vi "Lift Manager.vi"(1 "Setpoint":dbl) -> (0 "Current Height":dbl)   [LabVIEW 2014]
uses:
  <vilib>/Rock Robotics/Network Tables/SD Read Numeric Array.vi
  <vilib>/Rock Robotics/Network Tables/SD Write Boolean.vi
  <vilib>/addons/control/pid/pid.llb/PID (DBL).vi
  <vilib>/addons/control/pid/NI_PID_pid.lvlib
  <vilib>/ptbypt/NI_PtbyPt.lvlib
panel:
  out "Encoder Value":dbl
  in  "Zero Encoder":bool
  in  "Disabled?":bool=TRUE
  out "Motor":dbl
  out "Waveform Chart":cluster{"Distance":dbl, "output":dbl}(graph)
  in  "PID gains Down":T1={"proportional gain (Kc)"=2.0, "integral time (Ti, min)"=0.0, "derivative time (Td, min)"=0.0}
  in  "PID gains UP":T1={"proportional gain (Kc)"=2.0, "integral time (Ti, min)"=0.0, "derivative time (Td, min)"=0.0}
  # "Max: 24"
  # "Min: 8"
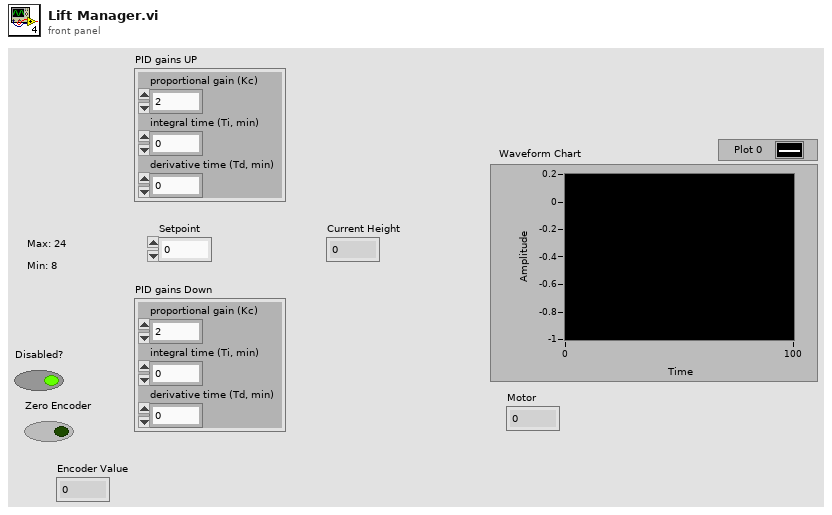
[diagram p1: front panel]
types:
  T1 = cluster{"proportional gain (Kc)":dbl, "integral time (Ti, min)":dbl, "derivative time (Td, min)":dbl}
  T2 = typedef "WPI_DigitalInputDevRef.ctl" = cluster{"DevStatus":errorcluster, "DIO Channel":T3, "Controller":T4}
  T3 = typedef "FPGA_DIOChannel.ctl" = enum8{"DIO 0", "DIO 1", "DIO 2", "DIO 3", "DIO 4", "DIO 5", "DIO 6", "DIO 7", "DIO 8", "DIO 9", "DIO MXP 0", "DIO MXP 1", "DIO MXP 2", "DIO MXP 3", "DIO MXP 4", "DIO MXP 5", "DIO MXP 6", "DIO MXP 7", "DIO MXP 8", "DIO MXP 9", "DIO MXP 10", "DIO MXP 11", "DIO MXP 12", "DIO MXP 13", "DIO MXP 14", "DIO MXP 15", "Invalid"}
  T4 = typedef "FPGA_TypedefDigitalModule.ctl" = enum16{"Controller 1"}
  T5 = typedef "WPI_EncoderDevRef.ctl" = cluster{"DevStatus":errorcluster, "EncoderIndex":T6, "CounterIndex":T7, "DistancePerCount":dbl, "Decoding Type":T8}
  T6 = typedef "FPGA_EncoderIdx.ctl" = enum8{"Enc 0", "Enc 1", "Enc 2", "Enc 3", "Enc 4", "Enc 5", "Enc 6", "Enc 7", "Invalid"}
  T7 = typedef "FPGA_CounterCtrSystemIndex.ctl" = enum8{"Ctr 0", "Ctr 1", "Ctr 2", "Ctr 3", "Ctr 4", "Ctr 5", "Ctr 6", "Ctr 7", "Invalid"}
  T8 = typedef "WPI_EncoderType.ctl" = enum16{"1x", "2x", "4x"}
  T9 = typedef "WPI_MotorControlDeviceRef.ctl" = cluster{"DeviceStatus":errorcluster, "Type":T10, "PWM":cluster{"Controller":T4, "PWM Channel":T11, "DeadBand":T12}, "CAN":cluster{"Device Number":u8, "Control Mode":T13, "Semaphore":T14, "Max Vout":dbl, "TalonSRX Control Mode":T15}, "Invert":bool, "TransformRef":T16, "InvTransformRef":T16}
  T10 = typedef "WPI_MotorControlType.ctl" = enum16{"PWM", "CAN", "CANTalonSRX"}
  T11 = typedef "FPGA_DIOPWMChannel.ctl" = enum8{"PWM 0", "PWM 1", "PWM 2", "PWM 3", "PWM 4", "PWM 5", "PWM 6", "PWM 7", "PWM 8", "PWM 9", "PWM MXP 0", "PWM MXP 1", "PWM MXP 2", "PWM MXP 3", "PWM MXP 4", "PWM MXP 5", "PWM MXP 6", "PWM MXP 7", "PWM MXP 8", "PWM MXP 9", "Invalid"}
  T12 = typedef "WPI_PWMDeadband.ctl" = cluster{"Name":string, "maxPositivePwm":i32, "minPositivePwm":i32, "centerPwm":i32, "maxNegativePwm":i32, "minNegativePwm":i32, "angularRange":u16}
  T13 = typedef "WPI_CANJaguar_ControlMode.ctl" = enum8{"Percent VBus", "Current", "Speed", "Position", "Voltage"}
  T14 = typedef "Semaphore RefNum" = refnum<k1>
  T15 = typedef "WPI_CANTalonSRX_APIControlMode.ctl" = enum8{"Percent VBus", "Speed", "Position", "Slave", "Unchanged / Invalid"}
  T16 = typedef "WPI_PWMTransform_ConPane.ctl" = refnum<vi>
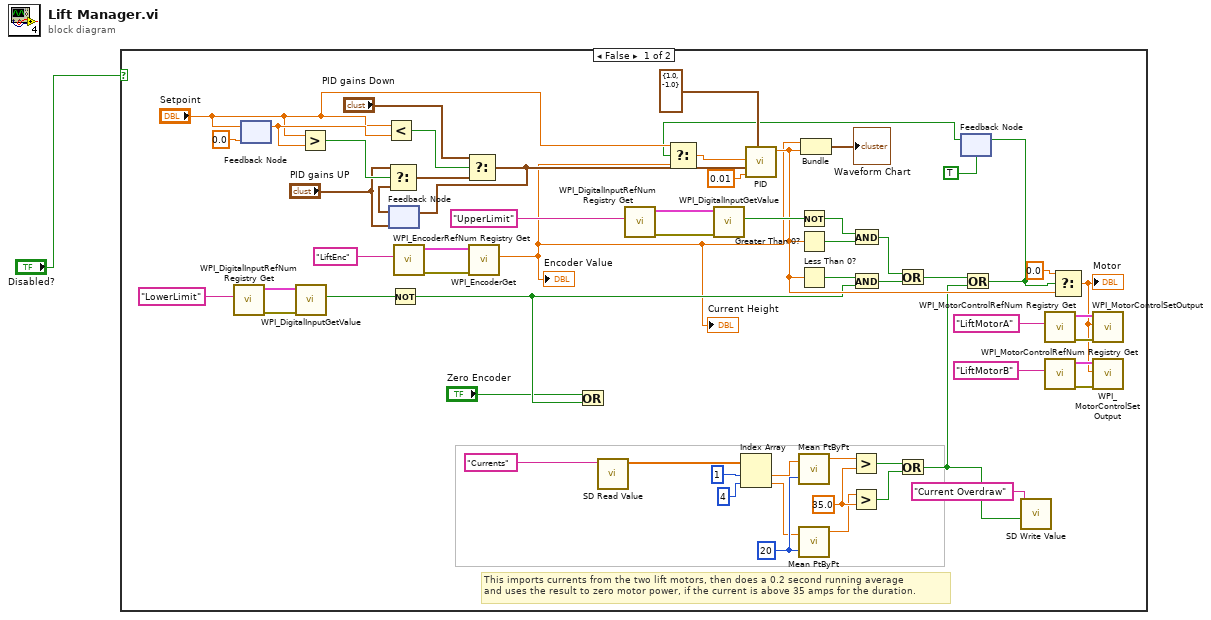
[diagram p0: block diagram]
diagram:
  n1 = case shown="False" "Disabled?" {
    frame False {
      w14 = 35.0
      w17 = 20 ("sample length")
      # "This imports currents from the two lift motors, then does a 0.2 second running average\nand uses the result to zero motor power, if the current is above 35 amps for the duration."
      n2 = call <vilib>:"WPI_DigitalInputRefNum Registry Get.vi"("refnum name"="LowerLimit") -> ("error out"=w44:errorcluster, "DigitalInputDevRef"=w43:T2)  [unwired: 9 in]
      n3 = feedback #1(0.0) -> (w60:dbl)
      n4 = feedback-in #1("Setpoint") -> ()
      n5 = call <vilib>:"WPI_DigitalInputGetValue.vi"("error in (no error)"=w44, "DigitalInputDevRef"=w43) -> ("Value"=w29:bool)  [unwired: 7 in, 2 out]
      n6 = Greater?(x="Setpoint", y=w60) -> (0:w59:bool)
      n7 = Less?(x="Setpoint", y=w60) -> (x < y?=w54:bool)
      n8 = feedback #2("PID gains UP") -> (w55:T1)
      n9 = Select(t="PID gains UP", s=w59, f=w55) -> (s? t:f=w56:T1)
      n10 = Not(x=w29) -> (.not. x?=w23:bool)
      n11 = call <vilib>:"WPI_EncoderRefNum Registry Get.vi"("refnum name"="LiftEnc") -> ("error out"=w51:errorcluster, "EncoderDevRef"=w50:T5)  [unwired: 9 in]
      n12 = Select(t="PID gains Down", s=w54, f=w56) -> (s? t:f=w53:T1)
      n13 = feedback-in #2(w53) -> ()
      n14 = call <vilib>:"WPI_EncoderGet.vi"("error in (no error)"=w51, "EncoderDevRef"=w50) -> ("Distance"=w5:dbl)  [unwired: 4 in, 5 out]
      "Current Height" <- w5
      "Encoder Value" <- w5
      n15 = Or(x="Zero Encoder", y=w23) -> ()  [unwired: 1 out]
      n16 = call-poly <vilib>:"SD Read Value.vi"("Name"="Currents") -> ("Numeric Array"=w20:dbl[])  [unwired: 8 in, 2 out]
      n17 = call <vilib>:"WPI_DigitalInputRefNum Registry Get.vi"("refnum name"="UpperLimit") -> ("error out"=w46:errorcluster, "DigitalInputDevRef"=w45:T2)  [unwired: 9 in]
      n18 = call <vilib>:"WPI_DigitalInputGetValue.vi"("error in (no error)"=w46, "DigitalInputDevRef"=w45) -> ("Value"=w28:bool)  [unwired: 7 in, 2 out]
      n19 = Index Array(array=w20, index #1=1 ("index"), index #2=4 ("index")) -> (element #1=w15:dbl, element #2=w16:dbl)
      n20 = Not(x=w28) -> (.not. x?=w27:bool)
      n21 = call <vilib>:"Mean PtByPt.vi"("x"=w15, "sample length"=w17) -> ("mean"=w12:dbl)  [unwired: 2 in, 1 out]
      n22 = call <vilib>:"Mean PtByPt.vi"("x"=w16, "sample length"=w17) -> ("mean"=w13:dbl)  [unwired: 2 in, 1 out]
      n23 = Greater?(x=w12, y=w14) -> (0:w10:bool)
      n24 = Greater?(x=w13, y=w14) -> (0:w11:bool)
      n25 = Or(x=w10, y=w11) -> (x .or. y?=w9:bool)
      n26 = feedback #3(TRUE) -> (w3:bool)
      n27 = Select(t="Setpoint", s=w3, f=w5) -> (s? t:f=w7:dbl)
      n28 = call-poly <vilib>:"PID.vi"("output range"=cluster{"output high":dbl, "output low":dbl} {"output high"=1.0, "output low"=-1.0}, "dt (s)"=0.01, "PID gains"=w53, "process variable"=w7) -> ("output"=w26:dbl)  [unwired: 6 in, 1 out]
      n29 = Greater Than 0?(x=w26) -> (x > 0?=w42:bool)
      n30 = Less Than 0?(x=w26) -> (x < 0?=w41:bool)
      n31 = Bundle("Distance"=w5, "output"=w26) -> (→"Waveform Chart":cluster{"Distance":dbl, "output":dbl})  [unwired: 1 in]
      n32 = And(x=w27, y=w42) -> (x .and. y?=w40:bool)
      n33 = And(x=w41, y=w23) -> (x .and. y?=w39:bool)
      n34 = Or(x=w40, y=w39) -> (x .or. y?=w38:bool)
      n35 = Or(x=w38, y=w9) -> (x .or. y?=w4:bool)
      n36 = feedback-in #3(w4) -> ()
      n37 = call-poly <vilib>:"SD Write Value.vi"("Boolean"=w9, "Name"="Current Overdraw") -> ()  [unwired: 8 in, 2 out]
      n38 = call <vilib>:"WPI_MotorControlRefNum Registry Get.vi"("refnum name"="LiftMotorA") -> ("error out"=w34:errorcluster, "MotorControlDevRef"=w33:T9)  [unwired: 9 in]
      n39 = call <vilib>:"WPI_MotorControlRefNum Registry Get.vi"("refnum name"="LiftMotorB") -> ("error out"=w31:errorcluster, "MotorControlDevRef"=w30:T9)  [unwired: 9 in]
      n40 = Select(t=0.0, s=w4, f=w26) -> (s? t:f=w24:dbl)
      "Motor" <- w24
      n41 = call <vilib>:"WPI_MotorControlSetOutput.vi"("error in (no error)"=w34, "Output"=w24, "MotorControlDevRef"=w33) -> ()  [unwired: 6 in, 3 out]
      n42 = call <vilib>:"WPI_MotorControlSetOutput.vi"("error in (no error)"=w31, "Output"=w24, "MotorControlDevRef"=w30) -> ()  [unwired: 6 in, 3 out]
    }
    frame True {
    }
  }
